vi "Test Get Failed Items when no Fails.vi"(8 "error in (no error)":errorcluster, 11 "Result Model Result Recording Test in":refnum<class "Result Model Result Recording Test.lvclass">) -> (0 "error out":errorcluster, 3 "Result Model Result Recording Test out":refnum<class "Result Model Result Recording Test.lvclass">)   [LabVIEW 2020, in "Result Model Result Recording Test.lvclass"]
uses:
  Result Model Result Recording Test.lvclass
  C:/Program Files (x86)/National Instruments/LabVIEW 2020/vi.lib/Astemes/LUnit/Test Case.lvclass
  Core/Result/Result.ctl
  Core/Result/Status.ctl
  Core/Result/Type.ctl
  Framework/Result Model/Tree Item Filter.ctl
  <vilib>/Astemes/LUnit/Test Case.lvclass/Test Case.ctl
  ae2c71b8-32bb-49d1-8500-0119bfec74ff.vi
  <vilib>/Astemes/LUnit/Palette/Pass.vi
  <vilib>/Astemes/LUnit/Palette/Fail.vi
  <vilib>/Astemes/LUnit/Compare Variants.vi
  <vilib>/Astemes/LUnit/Describe Comparison.vi
  <vilib>/Astemes/LUnit/Set Assertion Type.vi
  <vilib>/Astemes/LUnit/Add test result.vi
  <vilib>/Astemes/LUnit/Variant to string.vi
  <vilib>/Astemes/LUnit/LUnit Record Assertion Result.vi
  <vilib>/Astemes/LUnit/LUnit Aggregate Assertion Results.vi
  <vilib>/Astemes/LUnit/Method Result/LUnit Merge Status.vi
  <vilib>/Astemes/LUnit/LUnit Concatenate result strings.vi
  <vilib>/Utility/Data Type/Get Type Information.vi
  <vilib>/Utility/LVClass/Get LV Class Name.vi
  Framework/Result Model/Result Model.lvclass
  Core/Result/Result.lvlib
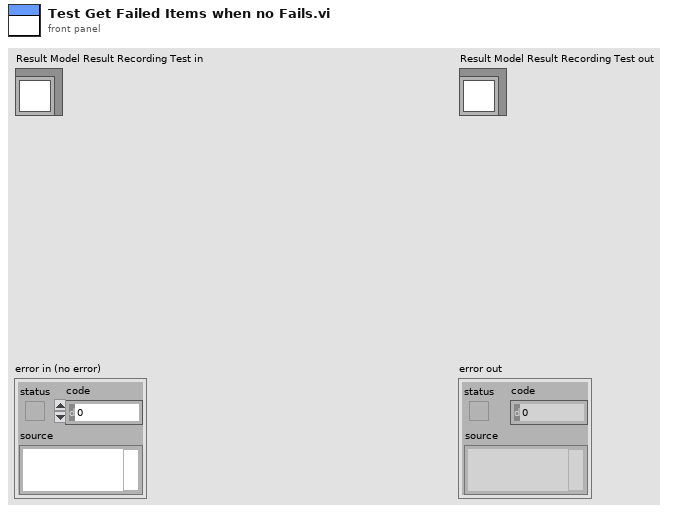
[diagram p1: front panel]
types:
  T1 = typedef "Result Model.lvclass/Tree Item Filter.ctl" = enum16{"All", "Only Fails"}
  T2 = typedef "Result.lvlib/Result.ctl" = cluster{"Name":string, "Message":string, "Description":string, "Status":T3, "Result Type":T4, "Execution Time":dbl}
  T3 = typedef "Result.lvlib/Status.ctl" = enum16{"", "Passed", "Failed", "Error", "Skipped", "Setup Error", "Broken", "Teardown Error"}
  T4 = typedef "Result.lvlib/Type.ctl" = enum16{"Method", "Case", "Suite", "Pass", "Fail", "Skip", "Pass if", "Fail if", "Pass if Error", "Fail if Error", "Pass if Equal", "Fail if Equal"}
  T5 = cluster{"Left Cell String":string, "Child Text":string[], "Child Tag":string, "Item Indent":i32, "Child Only?":bool, "Glyph Index":i32}[]
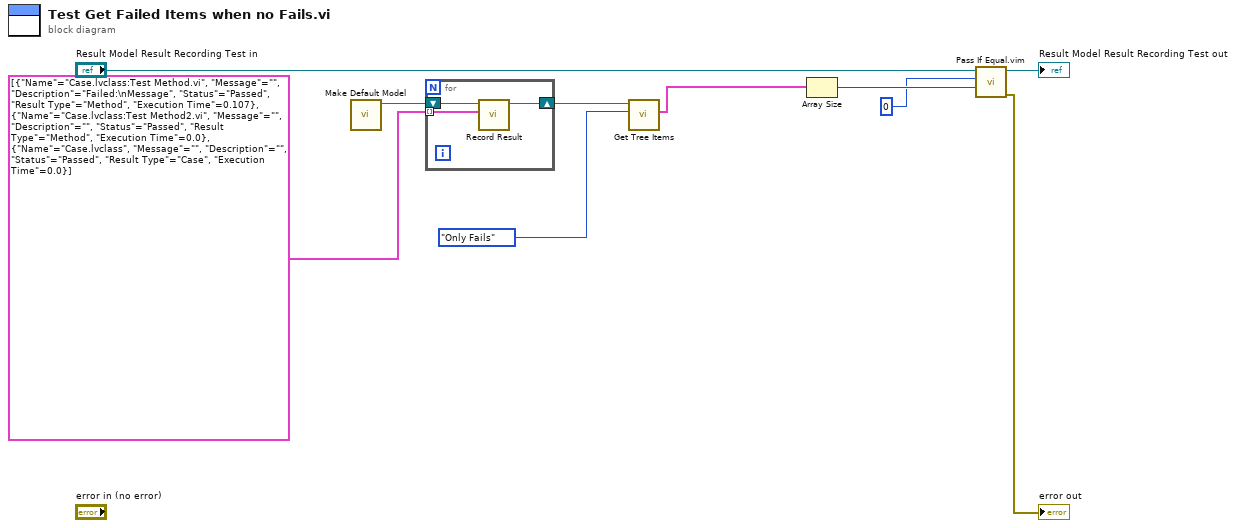
[diagram p0: block diagram]
diagram:
  n1 = call "Make Default Model.vi"() -> ("Result Model out"=w10:refnum<class "Result Model.lvclass">)  [unwired: 10 in, 1 out]
  n2 = for {
    tunnel: T2[] [{"Name"="Case.lvclass:Test Method.vi", "Message"="", "Description"="Failed:\nMessage", "Status"=enum."Passed", "Result Type"=enum."Method", "Execution Time"=0.107}, {"Name"="Case.lvclass:Test Method2.vi", "Message"="", "Description"="", "Status"=enum."Passed", "Result Type"=enum."Method", "Execution Time"=0.0}, {"Name"="Case.lvclass", "Message"="", "Description"="", "Status"=enum."Passed", "Result Type"=enum."Case", "Execution Time"=0.0}] ("Results") -> [w12] mode=indexing
    shift-right: [w11] -> w8
    shift-left: w10 -> [w13]
    n3 = call "Record Result.vi"("Results"=w12, "Result Model in"=w13) -> ("Result Model out"=w11:refnum<class "Result Model.lvclass">)  [unwired: 9 in]
  }
  n4 = call "Get Tree Items.vi"("Filter"=Tree_Item_Filter."Only Fails", "Result Model In"=w8) -> ("Tree Items"=w7:T5)  [unwired: 9 in]
  n5 = Array Size(array=w7) -> (size(s)=w3:i32)
  n6 = call "Pass If Equal.vim"("Actual"=w3, "Expected"=0 ("size(s)"), "LUnit Test Case In"="Result Model Result Recording Test in") -> ("error out"=→"error out":errorcluster, "LUnit Test Case Out"=→"Result Model Result Recording Test out":refnum<class "Result Model Result Recording Test.lvclass">)  [unwired: 7 in]
